vi "Finalize Data.vi"(8 "error in (no error)":errorcluster, 11 "Core Channel Configuration in":refnum<class "Core Channels Configuration.lvclass">) -> (0 "error out":errorcluster, 1 "data version":T1, 2 "data":string, 3 "Core Channel Configuration out":refnum<class "Core Channels Configuration.lvclass">)   [LabVIEW 2017, in "DSF Core.lvlib" / "Core Channels Configuration.lvclass"]
uses:
  Core Channels Configuration.lvclass
  C:/Git/DSF/Core/Classes/Configuration/Configuration.lvclass
  Typedefs/DSF Version Info.ctl
  Core Channels Configuration.lvclass/Core Channels Configuration.ctl
  Configuration.lvclass
  DSF Core.lvlib
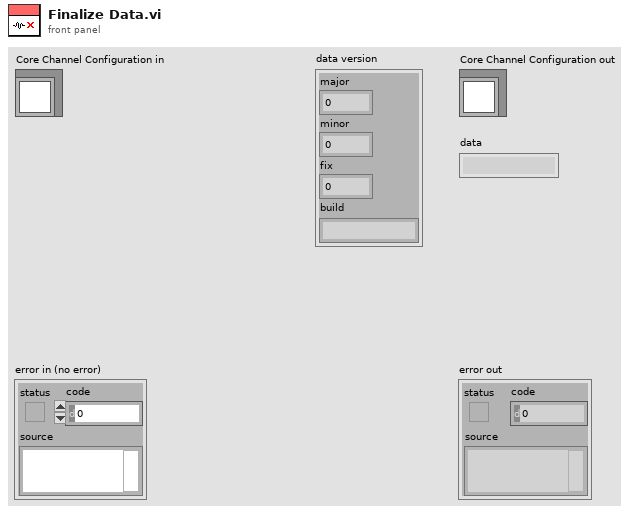
[diagram p1: front panel]
types:
  T1 = typedef "DSF Core.lvlib/DSF Version Info.ctl" = cluster{"major":i32, "minor":i32, "fix":i32, "build":string}
  T2 = typedef "DSF Core.lvlib/Core Channel Configuration.lvclass/Configuration.ctl" = cluster{"name":string, "units":string, "engine data type":T3, "string data type":T3, "string offset":u64}
  T3 = typedef "DSF Core.lvlib/DSF Data Type.ctl" = enum8{"Bool", "SGL", "DBL", "I8", "I16", "I32", "I64", "U8", "U16", "U32", "U64"}
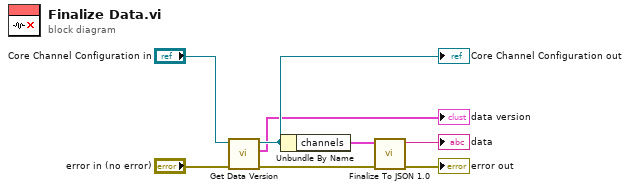
[diagram p0: block diagram]
diagram:
  n1 = call "Get Data Version.vi"("error in (no error)"="error in (no error)", "Configuration in"="Core Channel Configuration in") -> ("error out"=w5:errorcluster, "data version"=→"data version":T1, "Configuration out"=w3:refnum<class "Core Channels Configuration.lvclass">)  [unwired: 7 in]
  "Core Channel Configuration out" <- w3
  n2 = Unbundle By Name(w3) -> ("channels"=w8:T2[])
  n3 = call "Finalize To JSON 1.0.vi"("error in (no error)"=w5, "channel configuration 1.0"=w8) -> ("error out"=→"error out":errorcluster, "json"=→"data":string)  [unwired: 8 in]
